vi "Configure Automask.vi"(8 "error in (no error)":errorcluster, 9 "Mask Tolerance":T1 {"Units (0: Divisions)" items=["Divisions", "Volts/Time"]}, 10 "Source (1: Channel 1)":i32(ring) items=["Channel 1", "Channel 2", "Channel 3", "Channel 4"], 11 "VISA resource name":refnum<visa-resource-name>) -> (0 "error out":errorcluster, 3 "VISA resource name out":refnum<visa-resource-name>)   [LabVIEW 2009, in "Agilent 8000 Series.lvlib"]
doc: "Configures the Automask parameters."
uses:
  Agilent 8000 Series.lvlib
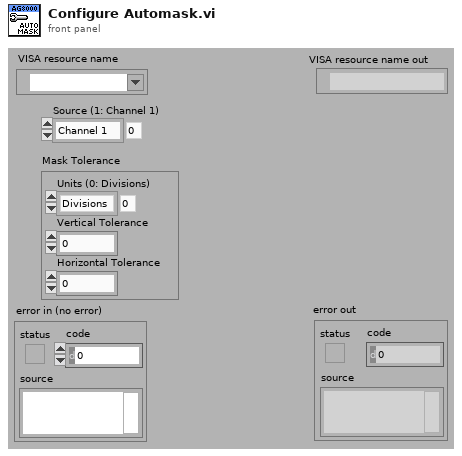
[diagram p1: front panel]
types:
  T1 = cluster{"Units (0: Divisions) ":i32, "Horizontal Tolerance":dbl, "Vertical Tolerance ":dbl}
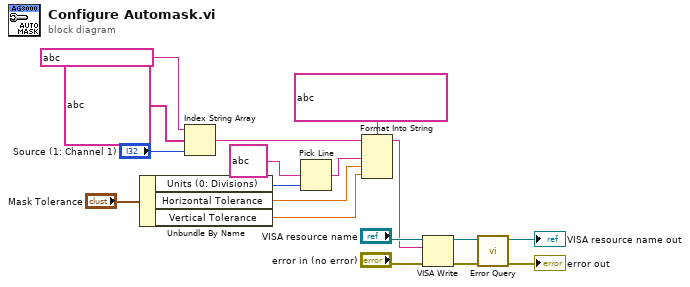
[diagram p0: block diagram]
diagram:
  n1 = Unbundle By Name("Mask Tolerance") -> ("Units (0: Divisions)"=w5:i32, "Horizontal Tolerance"=w8:dbl, "Vertical Tolerance"=w7:dbl)
  n2 = Index String Array(1:"Source (1: Channel 1)", 2:string[] ?, 3:string ? ("string (\"\")")) -> (0:w2:string)
  n3 = Pick Line(multi-line string=string ?, line index=w5) -> (output string=w3:string)  [unwired: 1 in]
  n4 = Format Into String(format string=string ?, initial string=w2, w3, w8, w7) -> (resulting string=w1:string)  [unwired: 1 in, 1 out]
  n5 = VISA Write(VISA resource name="VISA resource name", write buffer=w1, error in (no error)="error in (no error)") -> (VISA resource name out=w16:refnum<visa-resource-name>, error out=w15:errorcluster)  [unwired: 1 out]
  n6 = call "Error Query.vi"("error in (no error)"=w15, "VISA resource name"=w16) -> ("error out"=→"error out":errorcluster, "VISA resource name out"=→"VISA resource name out":refnum<visa-resource-name>)  [unwired: 6 in, 2 out]
